vi "Set SSR Status - Single.vi"(0 "reference in":refnum<class "SSR.lvclass">, 3 "SSR Channel Number (Zero Based)":i32, 4 "SSR Status to Set":bool, 5 "error in (no error)":errorcluster) -> (14 "reference out":refnum<class "SSR.lvclass">, 17 "SSR Channel Number (Zero Based) OUT":i32, 19 "error out":errorcluster)   [LabVIEW 2017, in "SSR.lvclass"]
uses:
  SSR.lvclass
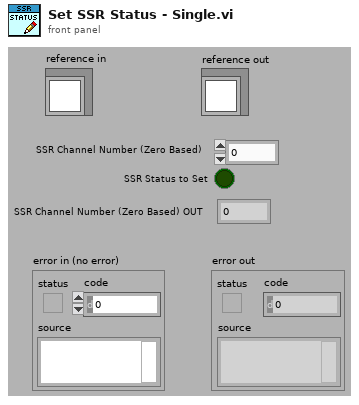
[diagram p1: front panel]
types:
  T1 = typedef "SSR.lvclass/ObjectAttributes.ctl" = cluster{"SSR Task":refnum<k21>, "SSR On/Off Status":bool, "Number of SSR Modules":u32, "Number of Total SSR Channels":u32, "SSR Module Names (NI-Max Name)":string[], "Number of Channels Per SSR Module":i32[], "SSR Status":bool[], "SSR Status to Set":bool[], "SSR VI Reference":refnum<vi>}
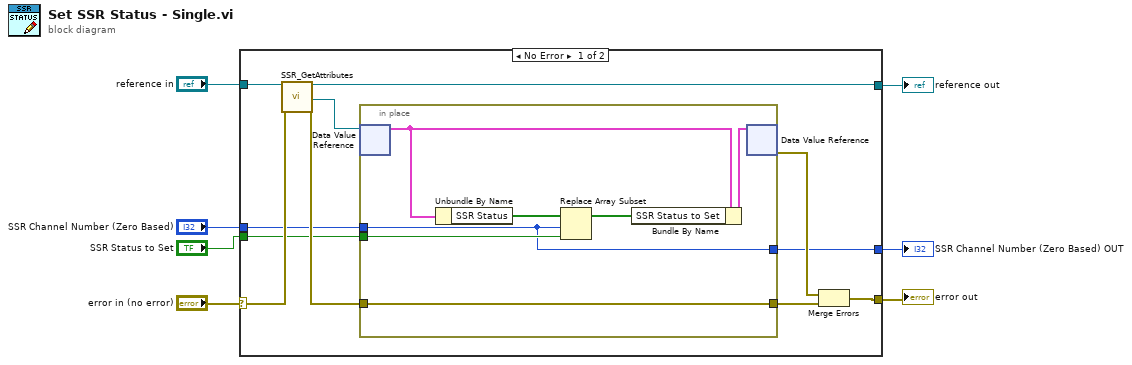
[diagram p0: block diagram]
diagram:
  n1 = case shown="No Error" "error in (no error)" {
    selector: "error in (no error)" -> [w17 w27]
    tunnel: [w14 w27] -> w6
    tunnel: [w15 w26] -> w4
    tunnel: "reference in" -> [w18 w26]
    tunnel: "SSR Channel Number (Zero Based)" -> [w10 _]
    tunnel: "SSR Status to Set" -> [w9 _]
    tunnel: [w8 _] -> w1
    frame No Error {
      n2 = call "SSR_GetAttributes.vi"("reference in"=w18, "error in (no error)"=w17) -> ("reference out"=w15:refnum<class "SSR.lvclass">, "DataRef"=w13:refnum<data-value>, "error out"=w12:errorcluster)  [unwired: 14 in, 1 out]
      n3 = in-place {
        in-place-border: w12 -> [w23]
        in-place-border: [w23] -> w11
        in-place-border: w10 -> [w19]
        in-place-border: w9 -> [w20]
        in-place-border: [w19] -> w8
        n4 = in-place-dvr #1(w13) -> (w24:T1)  [unwired: 1 out]
        n5 = Unbundle By Name(w24) -> ("SSR Status"=w22:bool[])
        n6 = Replace Array Subset(array=w22, new element=w20, index=w19) -> (w21:bool[])
        n7 = Bundle By Name(cluster=w24, "SSR Status to Set"=w21) -> (w25:T1)
        n8 = in-place-dvr #1(w25) -> (w16:errorcluster)  [unwired: 1 out]
      }
      n9 = Merge Errors(w16, w11) -> (w14:errorcluster)
    }
    frame Error {
    }
  }
  "error out" <- w6
  "reference out" <- w4
  "SSR Channel Number (Zero Based) OUT" <- w1
